vi "Non Linear PID Controller().vi"() -> (3 "Controller Library:Non Linear PID Controller.lvclass":refnum<class "Non Linear PID Controller.lvclass">)   [LabVIEW 2014, in "Controller Library.lvlib" / "Non Linear PID Controller.lvclass"]
uses:
  Non Linear PID Controller.lvclass
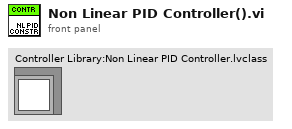
[diagram p1: front panel]
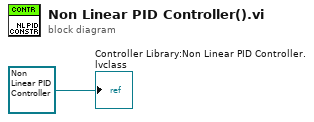
[diagram p0: block diagram]
diagram:
  "Controller Library:Non Linear PID Controller.lvclass" <- refnum<class "Non Linear PID Controller.lvclass"> refnum ("Controller Library:Non Linear PID Controller.lvclass")
